vi "Periodic Tasks.vi"(8 "error in":errorcluster) -> ()   [LabVIEW 2023]
doc: "This VI runs in parallel to other tasks. It can contain as many user-defined periodic loops as you need. These can carry out PID or other sorts of timed response."
uses:
  <vilib>/Rock Robotics/WPI/ThirdParty/Phoenix-LabVIEW/CANCoder/Controls/CTRE_Phoenix_CANcoder_Configurables.ctl
  <vilib>/Rock Robotics/WPI/ThirdParty/Phoenix-LabVIEW/CANCoder/Controls/CTRE_Phoenix_CANcoder_SensorInitializationStrategy.ctl
  <vilib>/Rock Robotics/WPI/ThirdParty/Phoenix-LabVIEW/CANCoder/Controls/CTRE_Phoenix_CANcoder_AbsoluteSensorRange.ctl
  <vilib>/Rock Robotics/WPI/ThirdParty/Phoenix-LabVIEW/Motor Controller/Controls/CTRE_Phoenix_MotorControl_VelocityMeasurementPeriod.ctl
  <vilib>/Rock Robotics/WPI/ThirdParty/Phoenix-LabVIEW/CANCoder/Controls/CTRE_Phoenix_CANcoder_SensorTimeBase.ctl
  <vilib>/Rock Robotics/WPI/DriverStation/WPI_DriverStationRobotMode2.ctl
  Robot Global Data.vi
  <vilib>/Rock Robotics/WPI/ThirdParty/Phoenix-LabVIEW/CANCoder/Get/CTRE_Phoenix_CANcoder_GetSensorData.vi
  <vilib>/Rock Robotics/WPI/ThirdParty/Phoenix-LabVIEW/Motor Controller/Get/CTRE_Phoenix_MotorController_GetGeneralStatus.vi
  <vilib>/Rock Robotics/WPI/ThirdParty/Phoenix-LabVIEW/Motor Controller/Get/CTRE_Phoenix_MotorController_GetSelectedSensorData.vi
panel:
  out "error out  3":errorcluster
  out "CANcoder Configurables":T1={"Sensor Initialization Strategy"=enum."Boot To Zero", "Absolute Sensor Range"=enum."Unsigned [0 to 360)", "Velocity Measurement Period"=100, "Velocity Measurement Window"=64, "Magnet Offset (Degrees)"=0.0, "Sensor Direction"=FALSE, "Sensor Coefficient"=0.087890625, "Unit String"="deg", "Sensor Time Base"=enum."PerMinute"} {"Velocity Measurement Period" items=["Period_1ms"=1, "Period_2ms"=2, "Period_5ms"=5, "Period_10ms"=10, "Period_20ms"=20, "Period_25ms"=25, "Period_50ms"=50, "Period_100ms"=100]; "Sensor Coefficient" format="%#_9g"}
  out "Absolute Position":dbl
  out "Velocity":dbl
  out "Position":dbl
  out "Velocity (Raw Sensor Units per 100 ms)":i32
  out "Position (Raw Sensor Units)":i32
  out "Device ID":i32
  out "Firmware Version":i32
  out "error out 2":errorcluster
  out "Sensor Position":dbl
  out "error out":errorcluster
  # "CANCODER"
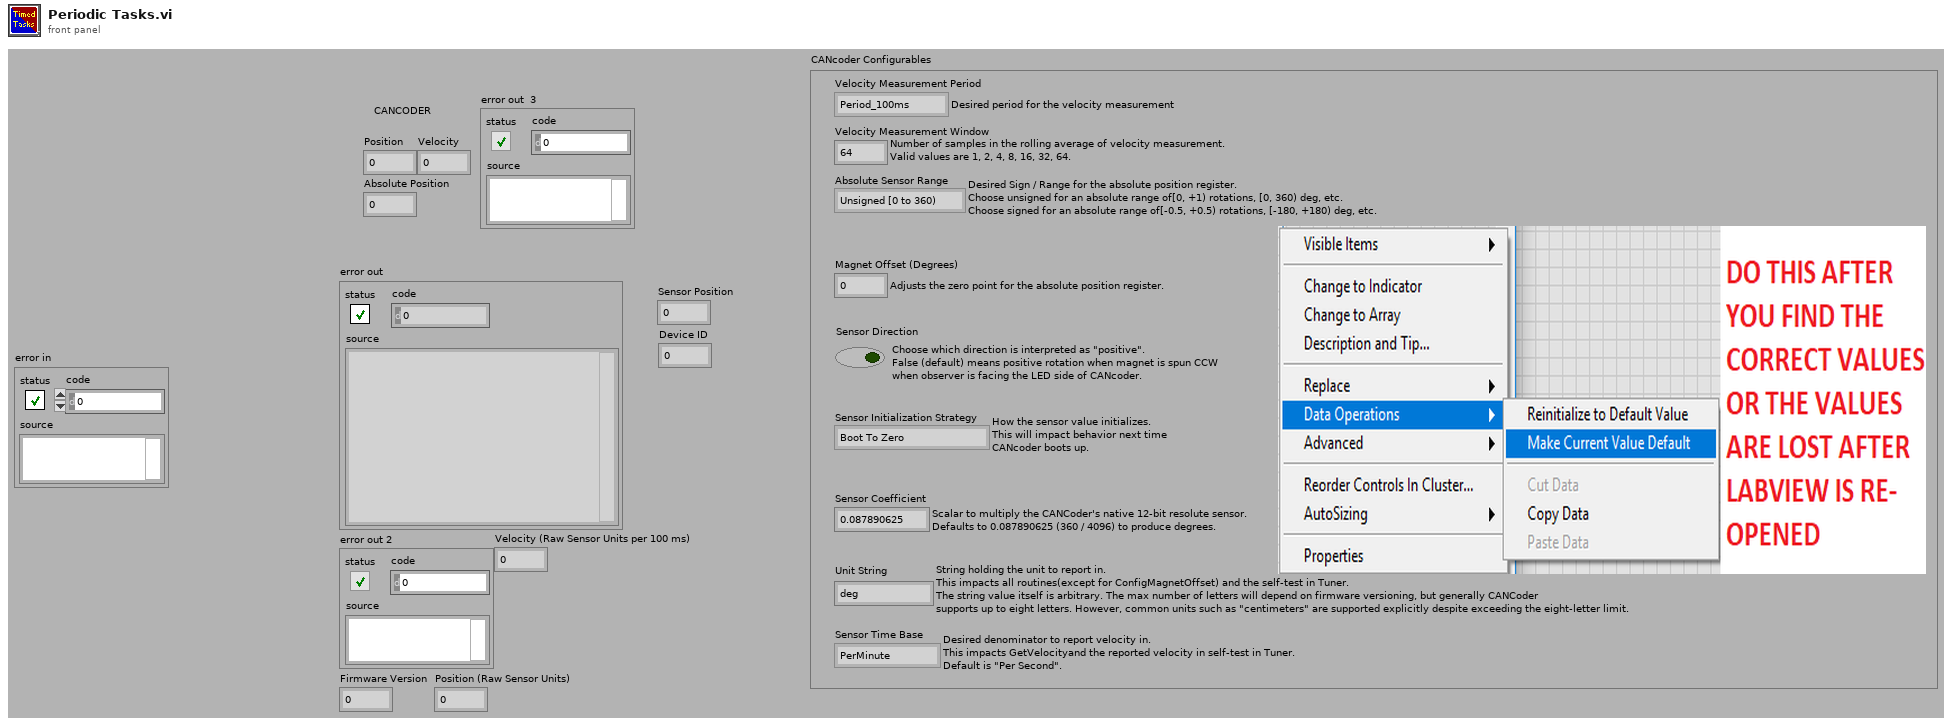
[diagram p1: front panel]
types:
  T1 = typedef "CTRE_Phoenix_CANcoder_Configurables.ctl" = cluster{"Sensor Initialization Strategy":T2, "Absolute Sensor Range":T3, "Velocity Measurement Period":T4, "Velocity Measurement Window":i32, "Magnet Offset (Degrees)":dbl, "Sensor Direction":bool, "Sensor Coefficient":dbl, "Unit String":string, "Sensor Time Base":T5}
  T2 = typedef "CTRE_Phoenix_CANcoder_SensorInitializationStrategy.ctl" = enum16{"Boot To Zero", "Boot To Absolute Position"}
  T3 = typedef "CTRE_Phoenix_CANcoder_AbsoluteSensorRange.ctl" = enum16{"Unsigned [0 to 360)", "Signed [-180 to +180)"}
  T4 = typedef "CTRE_Phoenix_MotorControl_VelocityMeasurementPeriod.ctl" = u16
  T5 = typedef "CTRE_Phoenix_CANcoder_SensorTimeBase.ctl" = enum16{"Per100Ms_Legacy", "PerSecond", "PerMinute"}
  T6 = typedef "WPI_DriverStationRobotMode2.ctl" = enum16{"Autonomous Disabled", "Autonomous Enabled", "Teleop Disabled", "Teleop Enabled", "Disconnected", "Finish", "Test Disabled", "Test Enabled", "Emergency Stopped"}
  T7 = typedef "WPI_MotorControlDeviceRef.ctl" = cluster{"DeviceStatus":errorcluster, "Type":T8, "PWM":cluster{"PWM Channel":T9, "DeadBand":T10}, "CAN":cluster{"Device Number":u8, "SetOutput VI Ref":variant, "GetOutput VI Ref":variant, "Enable VI Ref":variant, "Disable VI Ref":variant, "Data":variant}, "Invert":bool, "DIO PWM":cluster{"PWM \"Enable\" Channel":T9, "DIOChannel":T11, "PWM Rate":dbl}}
  T8 = typedef "WPI_MotorControlType.ctl" = enum16{"PWM", "CAN", "DIO PWM"}
  T9 = typedef "FPGA_DIOPWMChannel.ctl" = enum8{"PWM 0", "PWM 1", "PWM 2", "PWM 3", "PWM 4", "PWM 5", "PWM 6", "PWM 7", "PWM 8", "PWM 9", "PWM MXP 0", "PWM MXP 1", "PWM MXP 2", "PWM MXP 3", "PWM MXP 4", "PWM MXP 5", "PWM MXP 6", "PWM MXP 7", "PWM MXP 8", "PWM MXP 9", "Invalid"}
  T10 = typedef "WPI_PWMDeadband.ctl" = cluster{"Name":string, "maxPositivePwm":i32, "minPositivePwm":i32, "centerPwm":i32, "maxNegativePwm":i32, "minNegativePwm":i32, "angularRange":u16}
  T11 = typedef "FPGA_DIOChannel.ctl" = enum8{"DIO 0", "DIO 1", "DIO 2", "DIO 3", "DIO 4", "DIO 5", "DIO 6", "DIO 7", "DIO 8", "DIO 9", "DIO MXP 0", "DIO MXP 1", "DIO MXP 2", "DIO MXP 3", "DIO MXP 4", "DIO MXP 5", "DIO MXP 6", "DIO MXP 7", "DIO MXP 8", "DIO MXP 9", "DIO MXP 10", "DIO MXP 11", "DIO MXP 12", "DIO MXP 13", "DIO MXP 14", "DIO MXP 15", "SPI Port CS1", "SPI Port CS2", "SPI Port CS3", "SPI Port MISO", "SPI Port MOSI", "Invalid"}
  T12 = typedef "CTRE_Phoenix_CANcoder_DeviceRef.ctl" = cluster{"DeviceStatus":errorcluster, "Device Number":u8, "Handle":u64, "UsageFrame":u32, "Library Path":path}
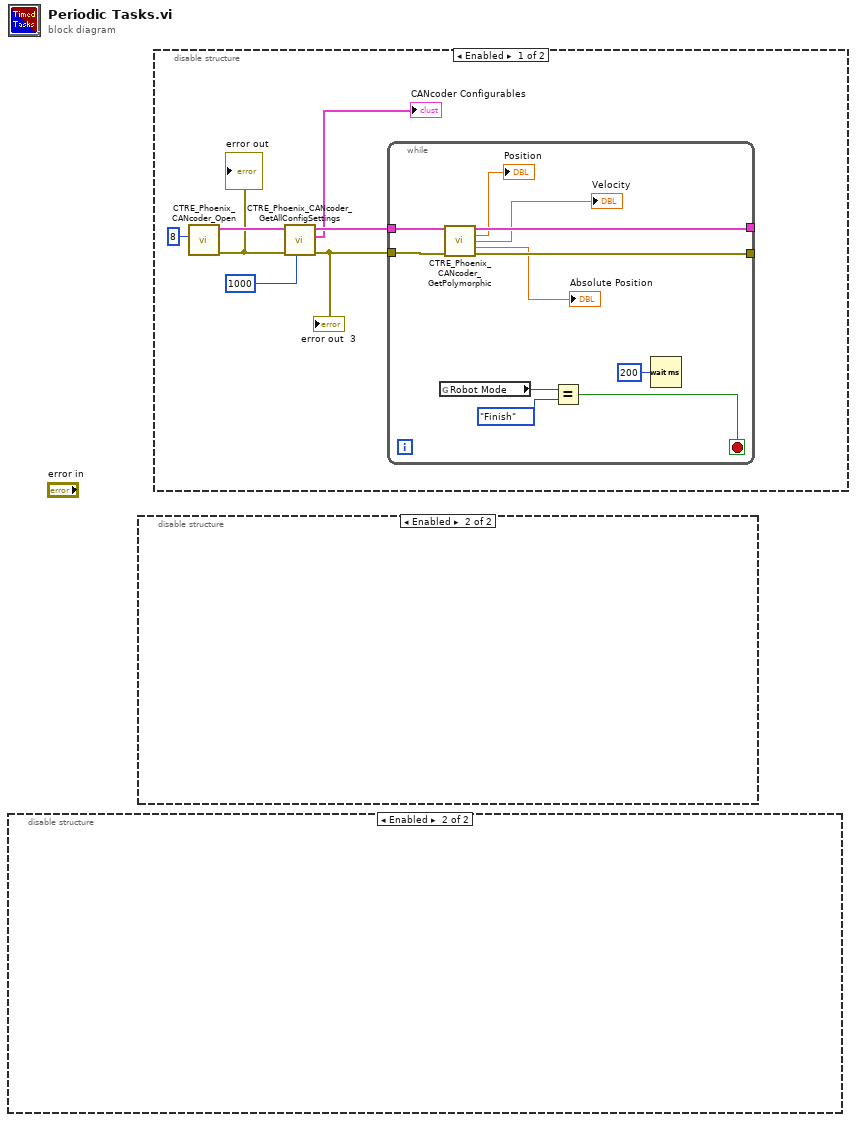
[diagram p0: block diagram]
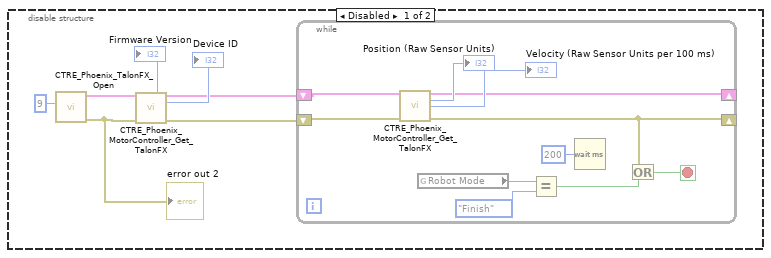
[diagram p2: hidden frame]
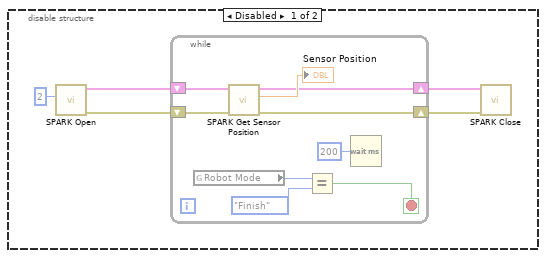
[diagram p3: hidden frame]
diagram:
  n1 = disable-structure shown="Enabled" {
    frame Disabled {
      n2 = call <vilib>:"CTRE_Phoenix_TalonFX_Open.vi"("Device Number"=u8 9) -> ("error out"=w1:errorcluster, "PhoenixMotorControlDevRef"=w4:T7)  [unwired: 9 in]
      "error out 2" <- w1
      n3 = call-poly <vilib>:"CTRE_Phoenix_MotorController_Get_TalonFX.vi"("PhoenixMotorControlDevRef"=w4, "error in"=w1) -> ("Firmware Version"=→"Firmware Version":i32, "PhoenixMotorControlDevRef"=w2:T7, "Device ID"=→"Device ID":i32, "error out"=w3:errorcluster)  [unwired: 8 in, 2 out]
      n4 = while {
        shift-right: [w15] -> _
        shift-left: w2 -> [w16]
        shift-right: [w10] -> _
        shift-left: w3 -> [w14]
        stop <- w8 stop-if-true
        n5 = call-poly <vilib>:"CTRE_Phoenix_MotorController_Get_TalonFX.vi"("PhoenixMotorControlDevRef"=w16, "error in"=w14) -> ("PhoenixMotorControlDevRef"=w15:T7, "Position (Raw Sensor Units)"=→"Position (Raw Sensor Units)":i32, "Velocity (Raw Sensor Units per 100 ms)"=→"Velocity (Raw Sensor Units per 100 ms)":i32, "error out"=w10:errorcluster)  [unwired: 10 in]
        n6 = global read "Robot Global Data.vi" "Robot Mode"() -> (w12:T6)
        n7 = Equal?(x=w12, y=WPI_DriverStationRobotMode2."Finish") -> (x = y?=w9:bool)
        n8 = Wait (ms)(milliseconds to wait=u32 200) -> ()  [unwired: 1 out]
        n9 = Or(x=w10, y=w9) -> (x .or. y?=w8:bool)
      }
    }
    frame Enabled {
    }
  }
  n10 = disable-structure shown="Enabled" {
    frame Disabled {
      n11 = call <vilib>:"SPARK Open.vi"("Device Number"=u8 2) -> ("error out"=w21:errorcluster, "MotorControlDeviceRef"=w22:T7)  [unwired: 9 in]
      n12 = while {
        shift-right: [w29] -> w20
        shift-left: w22 -> [w32]
        shift-right: [w28] -> w19
        shift-left: w21 -> [w30]
        stop <- w25 stop-if-true
        n13 = global read "Robot Global Data.vi" "Robot Mode"() -> (w26:T6)
        n14 = call <vilib>:"SPARK Get Sensor Position.vi"("error in (no error)"=w30, "MotorControlDevRef in"=w32) -> ("error out"=w28:errorcluster, "Sensor Position"=→"Sensor Position":dbl, "MotorControlDevRef out"=w29:T7)  [unwired: 6 in, 1 out]
        n15 = Equal?(x=w26, y=WPI_DriverStationRobotMode2."Finish") -> (x = y?=w25:bool)
        n16 = Wait (ms)(milliseconds to wait=u32 200) -> ()  [unwired: 1 out]
      }
      n17 = call <vilib>:"SPARK Close.vi"("error in"=w19, "MotorControlDeviceRef"=w20) -> ()  [unwired: 9 in, 1 out]
    }
    frame Enabled {
    }
  }
  n18 = disable-structure shown="Enabled" {
    frame Enabled {
      n19 = call <vilib>:"CTRE_Phoenix_CANcoder_Open.vi"("Device Number"=u8 8) -> ("error out"=w36:errorcluster, "CTRE_CANcoder_DeviceRef"=w38:T12)  [unwired: 9 in]
      "error out" <- w36
      n20 = call <vilib>:"CTRE_Phoenix_CANcoder_GetAllConfigSettings.vi"("timeoutMs"=1000, "error in (no error)"=w36, "CTRE_CANcoder_DeviceRef"=w38) -> ("error out"=w35:errorcluster, "CANcoder Configurables"=→"CANcoder Configurables":T1, "CTRE_CANcoder_DeviceRef"=w37:T12)  [unwired: 6 in]
      "error out  3" <- w35
      n21 = while {
        tunnel: w35 -> [w45]
        tunnel: w37 -> [w46]
        tunnel: [w44] -> _
        tunnel: [w43] -> _
        stop <- w48 stop-if-true
        n22 = global read "Robot Global Data.vi" "Robot Mode"() -> (w50:T6)
        n23 = call-poly <vilib>:"CTRE_Phoenix_CANcoder_GetPolymorphic.vi"("CTRE_CANcoder_DeviceRef"=w46, "error in"=w45) -> ("CTRE_CANcoder_DeviceRef"=w44:T12, "Position"=→"Position":dbl, "Velocity"=→"Velocity":dbl, "Absolute Position"=→"Absolute Position":dbl, "error out"=w43:errorcluster)  [unwired: 9 in]
        n24 = Equal?(x=w50, y=WPI_DriverStationRobotMode2."Finish") -> (x = y?=w48:bool)
        n25 = Wait (ms)(milliseconds to wait=u32 200) -> ()  [unwired: 1 out]
      }
    }
    frame Disabled {
    }
  }
